vi "Query Max Current Limit.vi"(8 "error in (no error)":errorcluster {"code" format="%.0x"}, 10 "Channel Name (1)":string="1", 11 "VISA resource name":refnum<visa-resource-name>) -> (0 "error out":errorcluster {"code" format="%.0x"}, 2 "Max Current Limit":dbl format="%^.3e", 3 "VISA resource name out":refnum<visa-resource-name>)   [LabVIEW 2018, in "Agilent N6700 Series.lvlib"]
doc: "Returns the maximum programmable current limit that the power supply accepts for a particular voltage level on a channel for the output range to which the power supply is currently configured."
uses:
  Agilent N6700 Series.lvlib
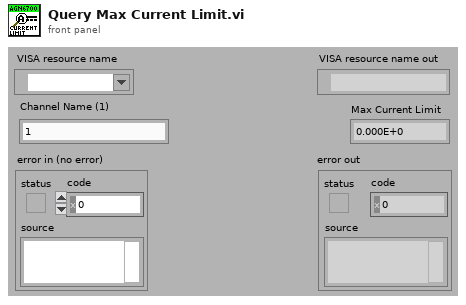
[diagram p1: front panel]
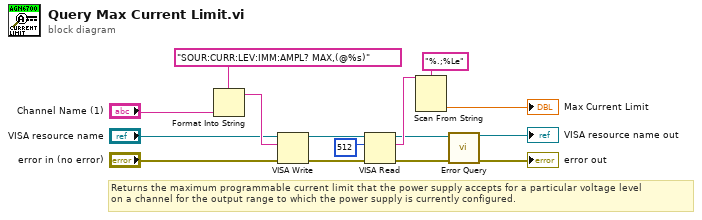
[diagram p0: block diagram]
diagram:
  # "Returns the maximum programmable current limit that the power supply accepts for a particular voltage level \non a channel for the output range to which the power supply is currently configured."
  n1 = Format Into String(format string="SOUR:CURR:LEV:IMM:AMPL? MAX,(@%s)", "Channel Name (1)") -> (resulting string=w8:string)  [unwired: 2 in, 1 out]
  n2 = VISA Write(VISA resource name="VISA resource name", write buffer=w8, error in (no error)="error in (no error)") -> (VISA resource name out=w14:refnum<visa-resource-name>, error out=w13:errorcluster)  [unwired: 1 out]
  n3 = VISA Read(VISA resource name=w14, byte count=u32 512, error in (no error)=w13) -> (VISA resource name out=w2:refnum<visa-resource-name>, read buffer=w12:string, error out=w1:errorcluster)  [unwired: 1 out]
  n4 = Scan From String(format string="%.;%Le", input string=w12) -> (output 1=→"Max Current Limit":dbl)  [unwired: 3 in, 3 out]
  n5 = call "Error Query.vi"("VISA resource name"=w2, "error in (no error)"=w1) -> ("VISA resource name out"=→"VISA resource name out":refnum<visa-resource-name>, "error out"=→"error out":errorcluster)  [unwired: 10 in, 2 out]
